vi "Trigger-Multirecord Acq.vi"(0 "niInstr Multirecord Acquisition Common v1 FPGA in":refnum<class "niInstr Multirecord Acquisition Common v1 FPGA.lvclass">, 1 "reset in":bool, 2 "Ch. correction output valid":bool, 3 "trigger data in":T3={"channel 0"=[0.0, 0.0], "channel 1"=[0.0, 0.0], "channel 2"=[0.0, 0.0], "channel 3"=[0.0, 0.0], "channel 4"=[0.0, 0.0], "channel 5"=[0.0, 0.0], "channel 6"=[0.0, 0.0], "channel 7"=[0.0, 0.0]}, 4 "data in":T2={"channel 0"=[0, 0], "channel 1"=[0, 0], "channel 2"=[0, 0], "channel 3"=[0, 0], "channel 4"=[0, 0], "channel 5"=[0, 0], "channel 6"=[0, 0], "channel 7"=[0, 0]}, 7 "overflow":bool, 8 "Trigger Settings":T1, 11 "trigger.rearm delay":u16, 13 "Trigger Data  input valid":bool) -> (14 "High":fxp<+/-,18,1>, 15 "Low":fxp<+/-,18,1>, 18 "TrigCount":u32, 19 "Trigger Index":u16)   [LabVIEW 2021]
uses:
  <instrlib>/_niInstr/Multirecord Acquisition/Common/v1/FPGA/niInstr Multirecord Acquisition Common v1 FPGA.lvclass
  C:/Program Files (x86)/National Instruments/LabVIEW 2021/instr.lib/_niInstr/Multirecord Acquisition/Interface/v1/FPGA/niInstr Multirecord Acquisition v1 FPGA.lvclass
  Custom Trigger Settings.ctl
  FPGA Interface Typedefinitions/Trigger Combination Type.ctl
  Trigger/SubVIs/Types/Trigger Type.ctl
  <instrlib>/_niInstr/Data Trigger/v1/Shared/Public/Level Configuration FXP(+-,18,1).ctl
  <instrlib>/_niInstr/Data Trigger/v1/Shared/Public/Level Configuration Trigger When.ctl
  <instrlib>/_niInstr/Data Trigger/v1/Shared/Public/Edge Configuration FXP(+-,18,1).ctl
  <instrlib>/_niInstr/Data Trigger/v1/Shared/Public/Edge Configuration Trigger Slope.ctl
  Update_Trigger_Center.ctl
  <instrlib>/_niInstr/Basic Elements/v1/FPGA/Private/Count Up U32.vi
  <instrlib>/_niInstr/Channel/v1/FPGA/Private/Select/Select FXP(+-,18,1,)xNspcx8ch.vi
  Trigger/Trigger FXP(+,-,18,1).vi
  <instrlib>/_niInstr/Channel/v1/FPGA/Private/Select and Interleave/Select And Interleave I16xNspcx8ch.vi
  <instrlib>/_niInstr/Multirecord Acquisition/Interface/v1/FPGA/Private/Write I16 Wrapper.vi
  <vilib>/rvi/FXPMathLib/FxpSub/XNode/nifxpmath_Sub.xnode
  <vilib>/rvi/FXPMathLib/FxpAdd/XNode/nifxpmath_Add.xnode
  <instrlib>/_niInstr/Multirecord Acquisition/Interface/v1/FPGA/niInstr Multirecord Acquisition v1 FPGA.lvclass
  <instrlib>/_niInstr/Channel/v1/FPGA/niInstr Channel v1 FPGA.lvlib
  FPGA Interface Typedefinitions/FPGA Interface Typedefinitions.lvlib
  <instrlib>/_niInstr/Data Trigger/v1/Shared/niInstr Data Trigger v1 Shared.lvlib
  <instrlib>/_niInstr/Basic Elements/v1/FPGA/niInstr Basic Elements v1 FPGA.lvlib
  <vilib>/rvi/FXPMathLib/sim/FxpSim.dll
  C:/Program Files (x86)/National Instruments/LabVIEW 2021/instr.lib/_niInstr/Multirecord Acquisition/Common/v1/FPGA/niInstr Multirecord Acquisition Common v1 FPGA.lvclass
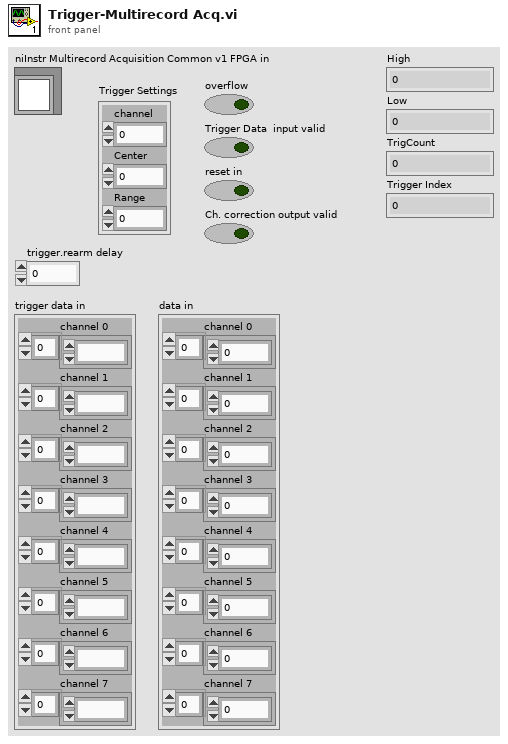
[diagram p1: front panel]
types:
  T1 = typedef "Custom Trigger Settings.ctl" = cluster{"channel":u8, "Center":fxp<+/-,24,1>, "Range":fxp<+,24,1>}
  T2 = cluster{"channel 0":i16[], "channel 1":i16[], "channel 2":i16[], "channel 3":i16[], "channel 4":i16[], "channel 5":i16[], "channel 6":i16[], "channel 7":i16[]}
  T3 = cluster{"channel 0":fxp<+/-,18,1>[], "channel 1":fxp<+/-,18,1>[], "channel 2":fxp<+/-,18,1>[], "channel 3":fxp<+/-,18,1>[], "channel 4":fxp<+/-,18,1>[], "channel 5":fxp<+/-,18,1>[], "channel 6":fxp<+/-,18,1>[], "channel 7":fxp<+/-,18,1>[]}
  T4 = typedef "Update_Trigger_Center.ctl" = cluster{"New Center":fxp<+/-,24,1>, "apply":bool}
  T5 = typedef "niInstr Data Trigger v1 Shared.lvlib/Level Configuration Trigger When.ctl" = enum8{"Trigger Above", "Trigger Below"}
  T6 = typedef "Trigger Type.ctl" = enum16{"Edge", "Level", "Custom"}
  T7 = typedef "niInstr Data Trigger v1 Shared.lvlib/Level Configuration FXP(+-,18,1).ctl" = cluster{"level":fxp<+/-,18,1>, "trigger when":T5}
  T8 = typedef "niInstr Data Trigger v1 Shared.lvlib/Edge Configuration FXP(+-,18,1).ctl" = cluster{"highLevel":fxp<+/-,18,1>, "lowLevel":fxp<+/-,18,1>, "trigger slope":T9}
  T9 = typedef "niInstr Data Trigger v1 Shared.lvlib/Edge Configuration Trigger Slope.ctl" = enum8{"Positive", "Negative"}
  T10 = typedef "FPGA Interface Typedefinitions.lvlib/Trigger Combination Type.ctl" = enum16{"Immediate", "A", "B", "OR", "AND", "A THEN B", "B THEN A", "High Resolution"}
  T11 = typedef "niInstr Multirecord Acquisition v1 FPGA.lvclass/Timestamp.ctl" = cluster{"timestamp":u64, "valid":bool}
  T12 = typedef "niInstr Types v1 Shared.lvlib/Input Triggers.ctl" = cluster{"start":bool, "advance":bool, "reference":bool, "start trigger index":u16, "advance trigger index":u16, "reference trigger index":u16, "reference trigger correction cycle count":u32}
  T13 = typedef "niInstr Types v1 Shared.lvlib/Sample Format.ctl" = cluster{"bits per channel":u16, "samples per clock":u16, "channels":u8}
  T14 = typedef "niInstr Multirecord Acquisition v1 FPGA.lvclass/Events.ctl" = cluster{"ready for start":bool, "ready for advance":bool, "ready for reference":bool, "end of record":bool, "done":bool, "start trigger":bool, "advance trigger":bool, "reference trigger":bool, "start trigger index":u16, "advance trigger index":u16, "reference trigger index":u16}
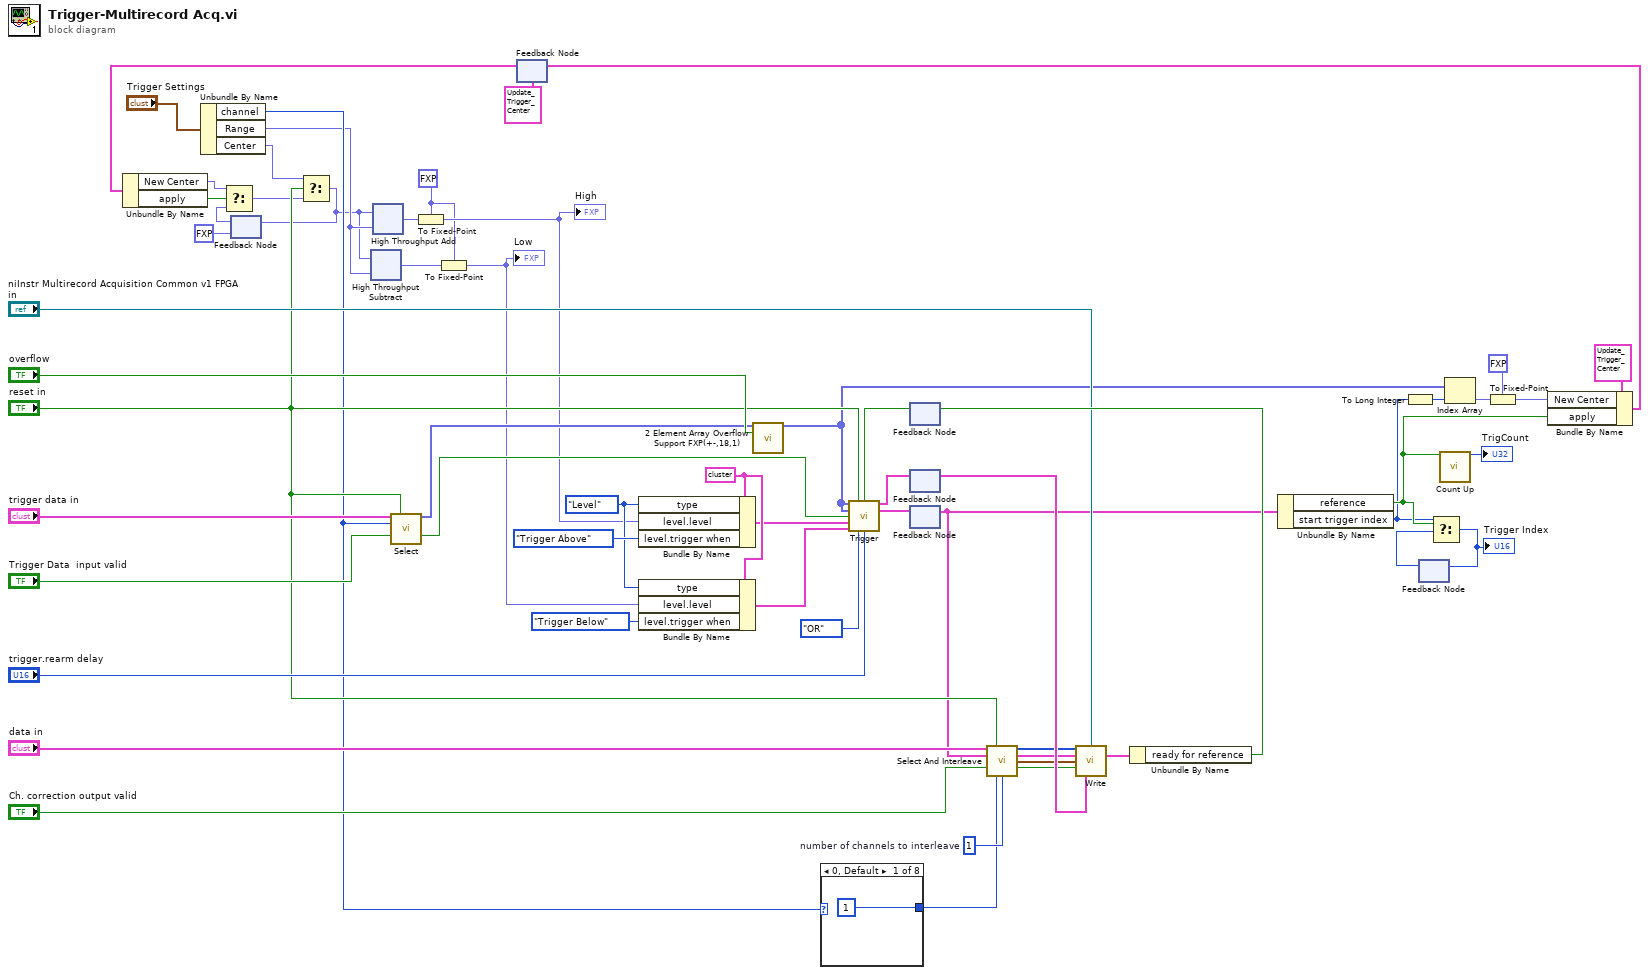
[diagram p0: block diagram]
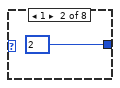
[diagram p2: hidden frame]
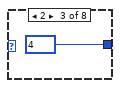
[diagram p3: hidden frame]
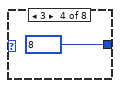
[diagram p4: hidden frame]
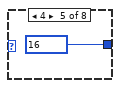
[diagram p5: hidden frame]
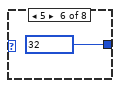
[diagram p6: hidden frame]
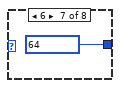
[diagram p7: hidden frame]
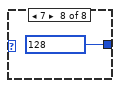
[diagram p8: hidden frame]
diagram:
  w2 = fxp<+/-,18,1> 0.0 ("StartCenter")
  w56 = Trigger_Type."Level" ("type")
  w59 = cluster{"type":T6, "level":T7, "edge":T8} {"type"=enum."Level", "level"={"level"=0.0, "trigger when"=enum."Trigger Above"}, "edge"={"highLevel"=0.0, "lowLevel"=0.0, "trigger slope"=enum."Positive"}} ("trigger.A")
  w54 = u8 1  # number of channels to interleave
  n1 = Unbundle By Name("Trigger Settings") -> ("channel"=w9:u8, "Range"=w6:fxp<+,24,1>, "Center"=w8:fxp<+/-,24,1>)
  n2 = feedback #1(fxp<+/-,24,1> 0.0 ("Center")) -> (w11:fxp<+/-,24,1>)
  n3 = call-poly <instrlib>:"Select.vi"("data in"="trigger data in", "reset"="reset in", "channel index"=w9, "input valid"="Trigger Data  input valid") -> ("channel out"=w43:fxp<+/-,18,1>[], "output valid"=w51:bool)  [unwired: 10 in]
  n4 = feedback #2(T4 {"New Center"=0.0, "apply"=FALSE}) -> (w14:T4)
  n5 = Unbundle By Name(w14) -> ("New Center"=w12:fxp<+/-,24,1>, "apply"=w13:bool)
  n6 = Select(t=w12, s=w13, f=w11) -> (s? t:f=w15:fxp<+/-,24,1>)
  n7 = Select(t=w8, s="reset in", f=w15) -> (s? t:f=w5:fxp<+/-,24,1>)
  n8 = feedback-in #1(w5) -> ()
  n9 = xnode ("High Throughput Subtract")("x"=w5, "y"=w6) -> ("x-y"=w7:fxp<+/-,26,3>)
  n10 = xnode ("High Throughput Add")("x"=w5, "y"=w6) -> ("x+y"=w4:fxp<+/-,26,3>)
  n11 = To Fixed-Point(fixed-point type=w2, number=w4) -> (fixed-point=w3:fxp<+/-,18,1>)
  "High" <- w3
  n12 = To Fixed-Point(fixed-point type=w2, number=w7) -> (fixed-point=w1:fxp<+/-,18,1>)
  "Low" <- w1
  n13 = Bundle By Name(cluster=w59, "type"=w56, "level.level"=w3, "level.trigger when"=Level_Configuration_Trigger_When."Trigger Above") -> (w41:cluster{"type":T6, "level":T7, "edge":T8})
  n14 = Bundle By Name(cluster=w59, "type"=w56, "level.level"=w1, "level.trigger when"=Level_Configuration_Trigger_When."Trigger Below") -> (w42:cluster{"type":T6, "level":T7, "edge":T8})
  n15 = call "2 Element Array Overflow Support FXP(+-,18,1).vi"("data in"=w43, "overflow"="overflow") -> ("data out"=w16:fxp<+/-,18,1>[])  [unwired: 13 in]
  n16 = case shown="0, Default" w9 {
    tunnel: [u16 1 ("channel.enable mask") u16 2 ("channel.enable mask") u16 4 ("channel.enable mask") u16 8 ("channel.enable mask") u16 16 ("channel.enable mask") u16 32 ("channel.enable mask") u16 64 ("channel.enable mask") u16 128 ("channel.enable mask")] -> w32
    frame 0, Default {
    }
    frame 1 {
    }
    frame 2 {
    }
    frame 3 {
    }
    frame 4 {
    }
    frame 5 {
    }
    frame 6 {
    }
    frame 7 {
    }
  }
  n17 = feedback #3() -> (w40:bool)  [unwired: 1 in]
  n18 = call-poly "Trigger.vi"("data A"=w16, "reset"="reset in", "trigger.ready for reference"=w40, "data B"=w16, "input valid"=w51, "trigger.A"=w41, "trigger.B"=w42, "trigger.combination type"=Trigger_Combination_Type."OR", "rearm delay"="trigger.rearm delay") -> ("timestamps"=w46:T11, "trigger.out"=w45:T12)  [unwired: 4 in, 1 out]
  n19 = feedback #4() -> (w47:T11)  [unwired: 1 in]
  n20 = feedback-in #4(w46) -> ()
  n21 = feedback #5() -> (w17:T12)  [unwired: 1 in]
  n22 = feedback-in #5(w45) -> ()
  n23 = call-poly <instrlib>:"Select And Interleave.vi"("data in"="data in", "reset"="reset in", "triggers in"=w17, "input valid"="Ch. correction output valid", "channel enable mask"=w32, "number of channels to interleave"=w54) -> ("interleaved data out"=w34:i16[], "triggers out"=w35:T12, "sample format out"=w36:T13, "output valid"=w37:bool)  [unwired: 5 in, 1 out]
  n24 = call-poly <instrlib>:"Write.vi"("data"=w34, "acquisition resources"="niInstr Multirecord Acquisition Common v1 FPGA in", "triggers"=w35, "sample format"=w36, "data valid"=w37, "timestamp"=w47) -> ("events"=w38:T14)  [unwired: 7 in, 2 out]
  n25 = Unbundle By Name(w38) -> ("ready for reference"=w39:bool)
  n26 = feedback-in #3(w39) -> ()
  n27 = Unbundle By Name(w17) -> ("reference"=w27:bool, "start trigger index"=w21:u16)
  n28 = To Long Integer(number=w21) -> (32bit integer=w22:i32)
  n29 = feedback #6() -> (w20:u16)  [unwired: 1 in]
  n30 = Select(t=w21, s=w27, f=w20) -> (s? t:f=w19:u16)
  "Trigger Index" <- w19
  n31 = feedback-in #6(w19) -> ()
  n32 = call-poly <instrlib>:"Count Up.vi"("increment"=w27) -> ("count out"=→"TrigCount":u32)  [unwired: 14 in]
  n33 = Index Array(array=w16, index=w22) -> (element=w23:fxp<+/-,18,1>)
  n34 = To Fixed-Point(fixed-point type=fxp<+/-,24,1> 0.0, number=w23) -> (fixed-point=w26:fxp<+/-,24,1>)
  n35 = Bundle By Name(cluster=T4 {"New Center"=0.0, "apply"=FALSE}, "New Center"=w26, "apply"=w27) -> (w28:T4)
  n36 = feedback-in #2(w28) -> ()
